vi "Set1DPlots.vi"(2 "1D graph":refnum<vi>, 3 "Axis for graph":i32, 4 "ScanCoords [mm]":T1) -> (0 "InitArray":dbl[](array[numeric]), 1 "PosArray":dbl[](array[numeric]))   [LabVIEW 2015]
panel:
  # "2D"
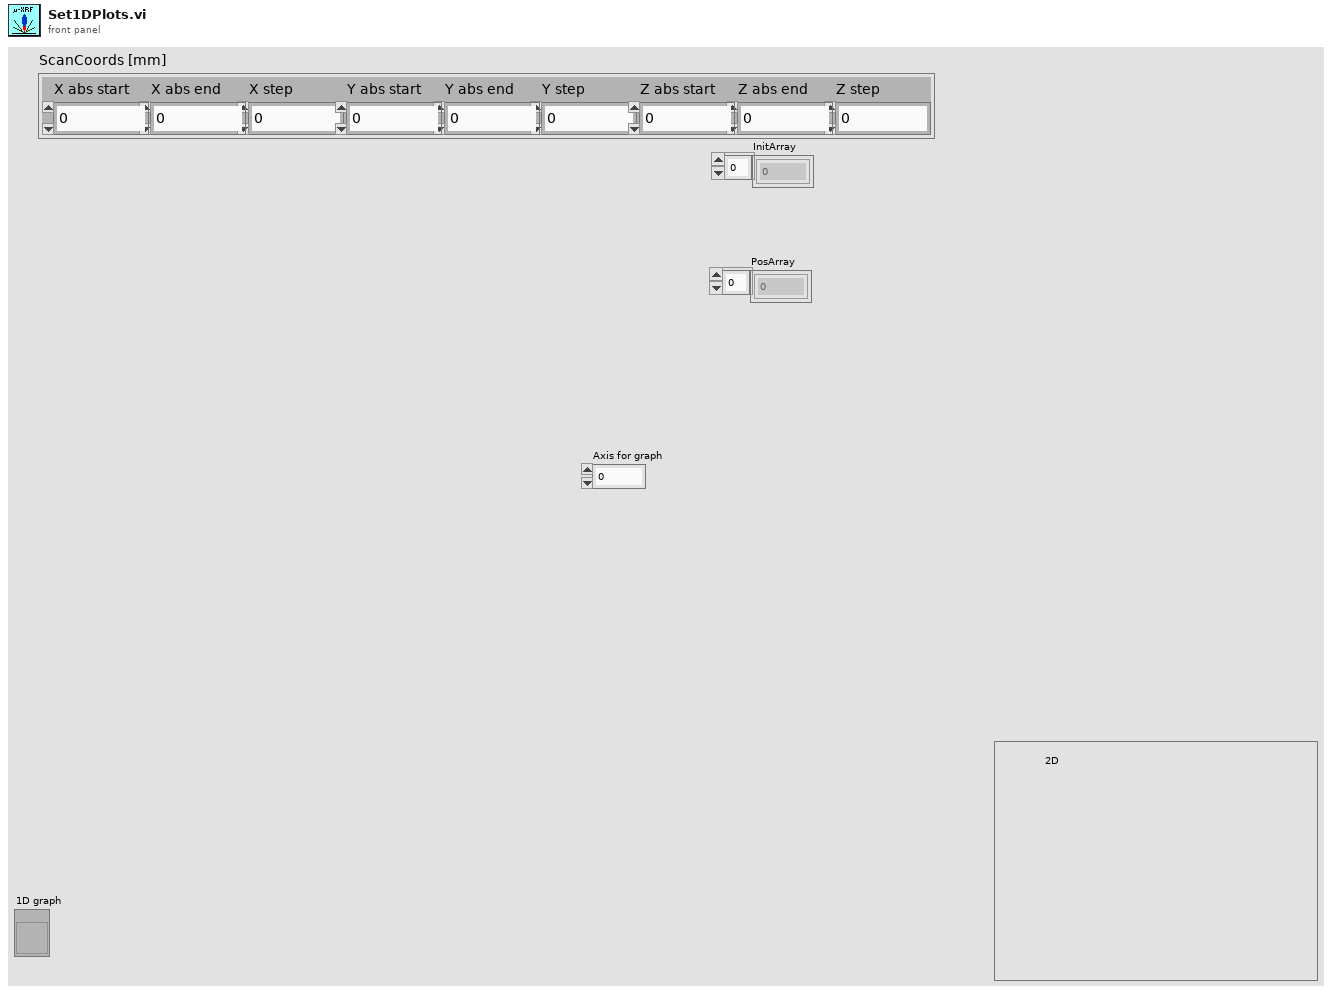
[diagram p1: front panel]
types:
  T1 = cluster{"X abs start":dbl, "X abs end":dbl, "Y abs start":dbl, "Y abs end":dbl, "Z abs start":dbl, "Z abs end":dbl, "X step":dbl, "Y step":dbl, "Z step":dbl}
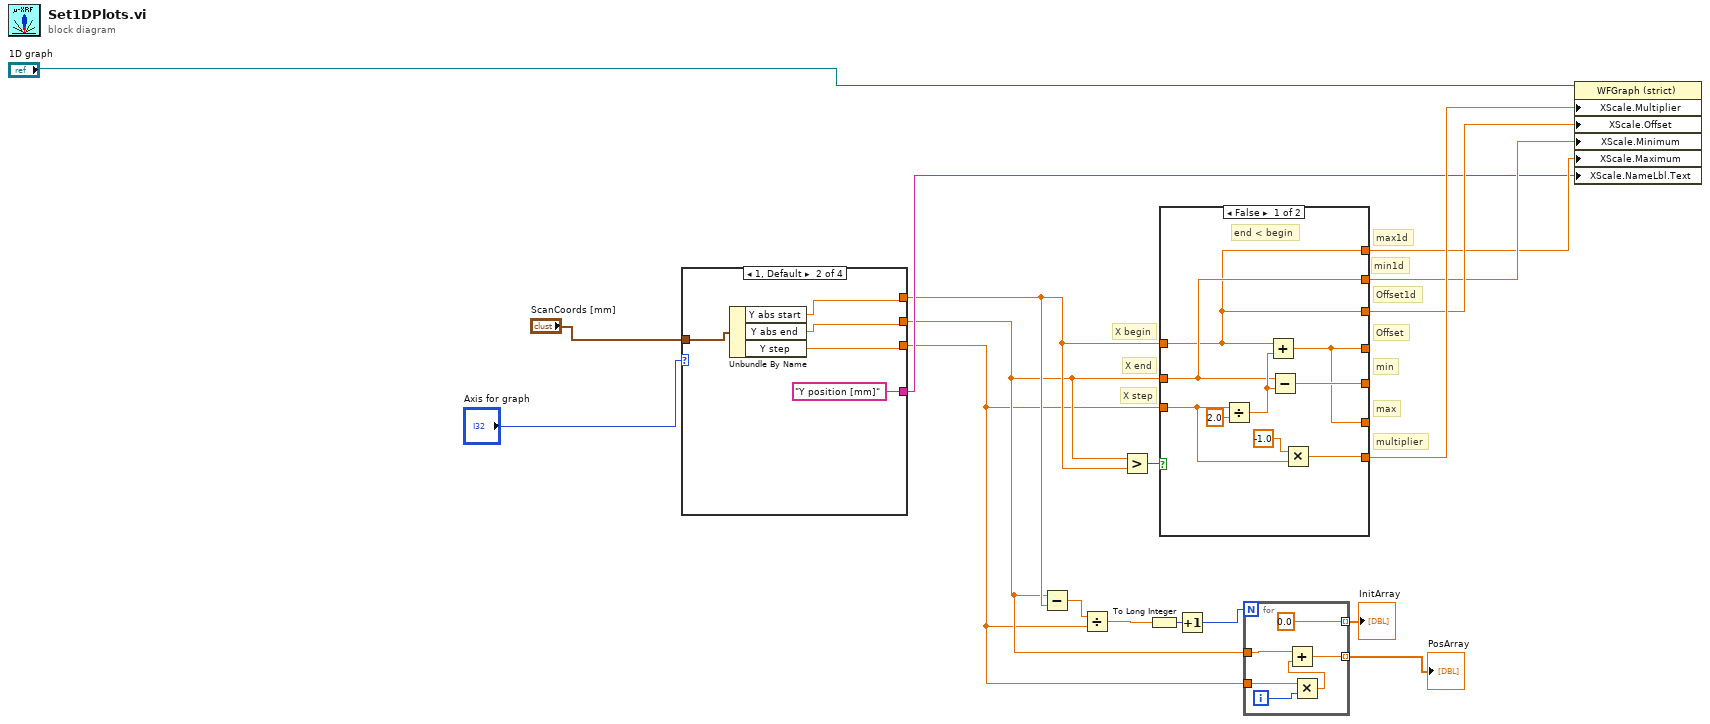
[diagram p0: block diagram]
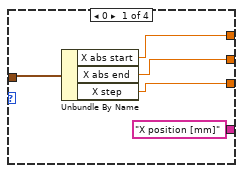
[diagram p2: hidden frame]
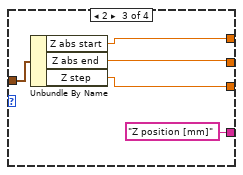
[diagram p3: hidden frame]
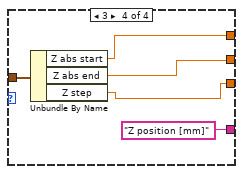
[diagram p4: hidden frame]
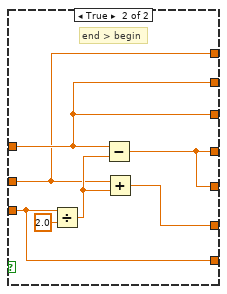
[diagram p5: hidden frame]
diagram:
  # "max1d"
  # "min1d"
  # "Offset1d"
  # "multiplier"
  # "min"
  # "max"
  # "Offset"
  # "X step"
  # "X end"
  # "X begin"
  n1 = case shown="1, Default" "Axis for graph" {
    tunnel: [w20 w25 w31 w35] -> w3
    tunnel: [w21 w26 w32 w36] -> w9
    tunnel: [w19 w24 w30 w34] -> w2
    tunnel: ["X position [mm]" "Y position [mm]" "Z position [mm]" "Z position [mm]"] -> w12
    tunnel: "ScanCoords [mm]" -> [w22 w27 w29 w37]
    frame 0 {
      n2 = Unbundle By Name(w22) -> ("X abs start"=w21:dbl, "X abs end"=w20:dbl, "X step"=w19:dbl)
    }
    frame 1, Default {
      n3 = Unbundle By Name(w27) -> ("Y abs start"=w26:dbl, "Y abs end"=w25:dbl, "Y step"=w24:dbl)
    }
    frame 2 {
      n4 = Unbundle By Name(w29) -> ("Z abs start"=w32:dbl, "Z abs end"=w31:dbl, "Z step"=w30:dbl)
    }
    frame 3 {
      n5 = Unbundle By Name(w37) -> ("Z abs start"=w36:dbl, "Z abs end"=w35:dbl, "Z step"=w34:dbl)
    }
  }
  n6 = Subtract(x=w3, y=w9) -> (x-y=w8:dbl)
  n7 = Divide(x=w8, y=w2) -> (x/y=w6:dbl)
  n8 = Greater?(x=w3, y=w9) -> (0:w17:bool)
  n9 = To Long Integer(number=w6) -> (32bit integer=w7:i32)
  n10 = case shown="False" w17 {
    tunnel: w9 -> [w39 w49]
    tunnel: w3 -> [w40 w48]
    tunnel: w2 -> [w45 w50]
    tunnel: [w41 w51] -> _
    tunnel: [w41 w52] -> _
    tunnel: [w42 w51] -> _
    tunnel: [w44 w50] -> w16
    tunnel: [w39 w49] -> w15
    tunnel: [w40 w49] -> w14
    tunnel: [w39 w48] -> w13
    frame False {
      # "end < begin"
      n11 = Divide(x=w45, y=2.0) -> (x/y=w43:dbl)
      n12 = Add(x=w39, y=w43) -> (x+y=w41:dbl)
      n13 = Subtract(x=w40, y=w43) -> (x-y=w42:dbl)
      n14 = Multiply(x=-1.0 ("t"), y=w45) -> (x*y=w44:dbl)
    }
    frame True {
      # "end > begin"
      n15 = Divide(x=w50, y=2.0) -> (x/y=w53:dbl)
      n16 = Subtract(x=w49, y=w53) -> (x-y=w51:dbl)
      n17 = Add(x=w48, y=w53) -> (x+y=w52:dbl)
    }
  }
  n18 = Increment(x=w7) -> (x+1=w5:i32)
  n19 = for {
    N: w5 -> [_]
    tunnel: [0.0] -> w4 mode=indexing
    tunnel: w3 -> [w59]
    tunnel: w2 -> [w58]
    tunnel: [w55] -> w1 mode=indexing
    i -> [w57]
    n20 = Multiply(x=w58, y=w57) -> (x*y=w56:dbl)
    n21 = Add(x=w59, y=w56) -> (x+y=w55:dbl)
  }
  "InitArray" <- w4
  "PosArray" <- w1
  n22 = property class="WFGraph (strict)"(reference="1D graph", "XScale.Multiplier"=w16, "XScale.Offset"=w15, "XScale.Minimum"=w14, "XScale.Maximum"=w13, "XScale.NameLbl.Text"=w12) -> ()  [unwired: 1 in, 2 out]
